vi "Return MutationCode Folder.vi"() -> (3 "Base Path Mutation Code":path)   [LabVIEW 2021, in "lv_icon.lvlib"]
uses:
  lv_icon.lvlib
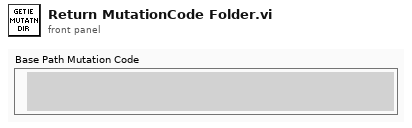
[diagram p1: front panel]
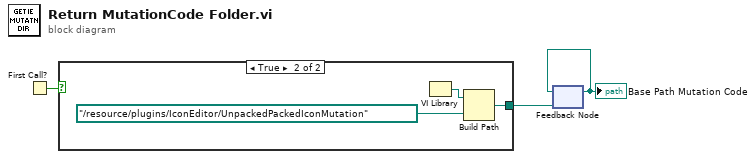
[diagram p0: block diagram]
diagram:
  n1 = First Call?() -> (First Call?: T/F=w1:bool)
  n2 = case shown="True" w1 {
    tunnel: [_ w6] -> w3
    frame False {
    }
    frame True {
      n3 = VI Library() -> (path=w5:path)
      n4 = Build Path(base path=w5, name or relative path=path "../resource/plugins/IconEditor/UnpackedPackedIconMutation" ("path")) -> (appended path=w6:path)
    }
  }
  n5 = feedback #1(w3) -> (w2:path)
  "Base Path Mutation Code" <- w2
  n6 = feedback-in #1(w2) -> ()
